vi "Generate Synchronous Strings For Moving Motors.vi"(7 "Motor List":u8[](array[numeric]), 8 "Error in (no error)":errorcluster, 9 "Dynamixel Speeds":u16[][](array[numeric]), 11 "Dynamixel Positions":u16[][](array[numeric])) -> (0 "Error out":errorcluster, 3 "Compiled Sync Parameters":string[](array[string]))   [LabVIEW 2016]
doc: "This VI combines the <B>Motor List</B> and corresponding positions and speeds in to sychronous write command. These commands when issues will move all of the motors at the same time."
uses:
  <instrlib>/Dynamixel Motor/Dynamixel Motor.lvlib
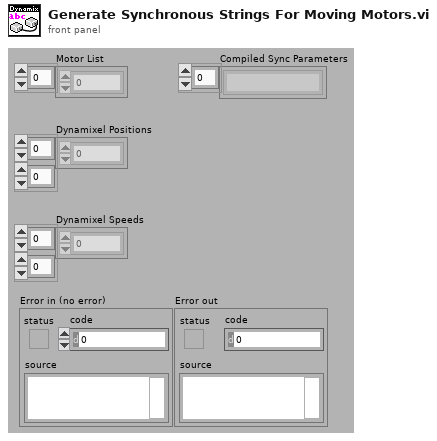
[diagram p1: front panel]
types:
  T1 = enum16{"big-endian, network order", "native, host order", "little-endian"}
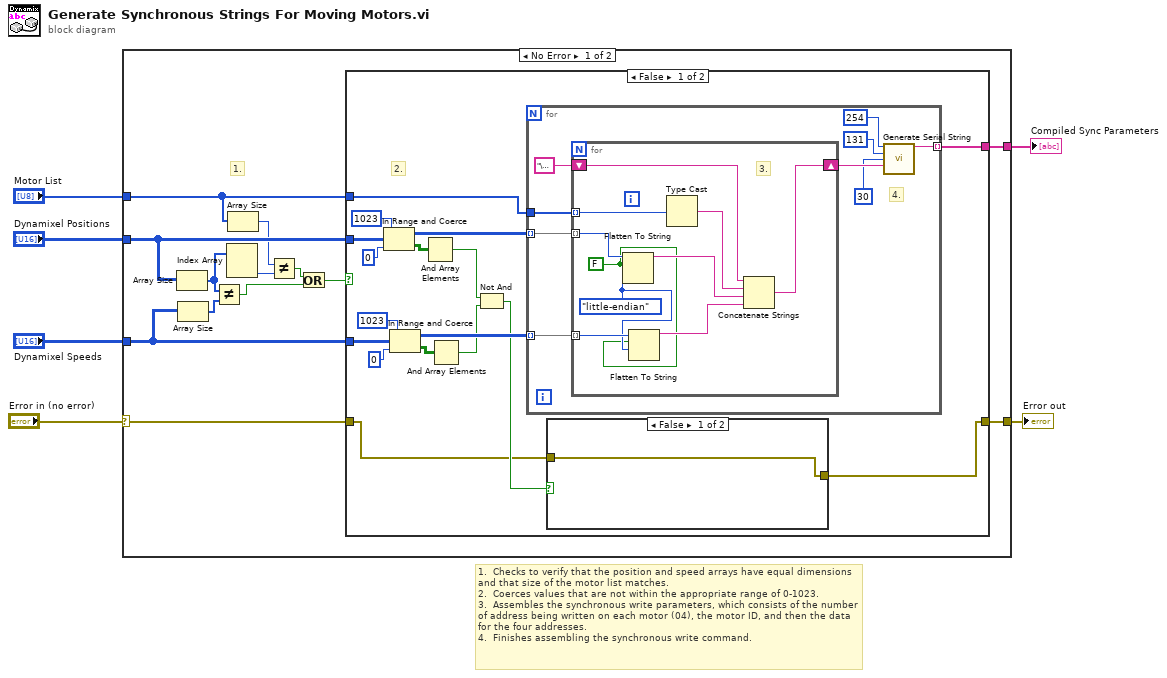
[diagram p0: block diagram]
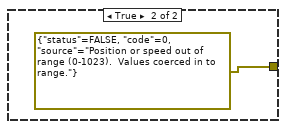
[diagram p2: hidden frame]
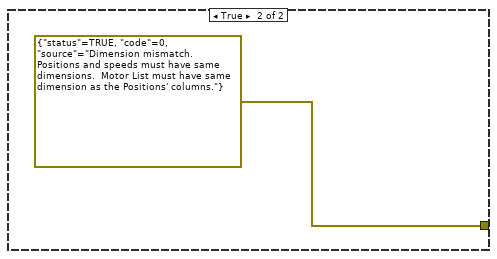
[diagram p3: hidden frame]
diagram:
  # "1.  Checks to verify that the position and speed arrays have equal dimensions \nand that size of the motor list matches.\n2.  Coerces values that are not within the appropriate range of 0-1023.\n3.  Assembles the synchronous write parameters, which consists of the number \nof address being written on each motor (04), the motor ID, and then the data \nfor the four addresses.\n4.  Finishes assembling the synchronous write command."
  n1 = case shown="No Error" "Error in (no error)" {
    selector: "Error in (no error)" -> [w7 w59]
    tunnel: [w19 _] -> w6
    tunnel: "Dynamixel Positions" -> [w18 _]
    tunnel: "Dynamixel Speeds" -> [w17 _]
    tunnel: "Motor List" -> [w15 _]
    tunnel: [w8 w59] -> w2
    frame No Error {
      # "1."
      n2 = Array Size(array=w18) -> (size(s)=w12:i32[])
      n3 = Array Size(array=w17) -> (size(s)=w16:i32[])
      n4 = Not Equal?(x=w12, y=w16) -> (x != y?=w13:bool)
      n5 = Index Array(array=w12) -> (element #2=w9:i32)  [unwired: 2 in, 1 out]
      n6 = Array Size(array=w15) -> (size(s)=w10:i32)
      n7 = Not Equal?(x=w10, y=w9) -> (x != y?=w11:bool)
      n8 = Or(x=w11, y=w13) -> (x .or. y?=w14:bool)
      n9 = case shown="False" w14 {
        tunnel: [w36 _] -> w19
        tunnel: w18 -> [w29 _]
        tunnel: w17 -> [w28 _]
        tunnel: w15 -> [w27 _]
        tunnel: [w20 errorcluster {"status"=TRUE, "code"=0, "source"="Dimension mismatch.  Positions and speeds must have same dimensions.  Motor List must have same dimension as the Positions' columns."} ("error in (no error)")] -> w8
        tunnel: w7 -> [w21 _]
        frame False {
          # "2."
          n10 = In Range and Coerce(upper limit=u16 1023, x=w29, lower limit=u16 0) -> (coerced(x)=w33:u16[][], In Range?=w25:bool[][])
          n11 = In Range and Coerce(upper limit=u16 1023, x=w28, lower limit=u16 0) -> (coerced(x)=w30:u16[][], In Range?=w26:bool[][])
          n12 = And Array Elements(Boolean array=w25) -> (logical AND=w23:bool)
          n13 = And Array Elements(Boolean array=w26) -> (logical AND=w24:bool)
          n14 = Not And(1:w24, 2:w23) -> (0:w22:bool)
          n15 = for {
            tunnel: w33 -> [w47] mode=indexing
            tunnel: w30 -> [w46] mode=indexing
            tunnel: [w42] -> w36 mode=indexing
            tunnel: w27 -> [w44]
            # "4."
            n16 = for {
              tunnel: w47 -> [w53] mode=indexing
              tunnel: w46 -> [w51] mode=indexing
              shift-right: [w57] -> w43
              shift-left: "\u0004" -> [w56]
              tunnel: w44 -> [w55] mode=indexing
              w49 = T1."little-endian" ("byte order (0:big-endian, network order)")
              w48 = FALSE ("prepend array or string size? (T)")
              # "3."
              n17 = Flatten To String(anything=w53, prepend array or string size? (T)=w48, byte order (0:big-endian, network order)=w49) -> (data string=w52:string)  [unwired: 1 in, 2 out]
              n18 = Flatten To String(anything=w51, prepend array or string size? (T)=w48, byte order (0:big-endian, network order)=w49) -> (data string=w50:string)  [unwired: 1 in, 2 out]
              n19 = Type Cast(x=w55) -> (*(type *) &x=w54:string)  [unwired: 1 in]
              n20 = Concatenate Strings(w56, w54, w52, w50) -> (w57:string)
            }
            n21 = call <instrlib>:"Generate Serial String.vi"("Motor ID"=u8 254 ("Motor ID (0)"), "Command"=u8 131 ("Motor ID (0)"), "Address"=u8 30 ("Motor ID (0)"), "Parameters"=w43) -> ("Command to Serial"=w42:string)  [unwired: 10 in, 1 out]
          }
          n22 = case shown="False" w22 {
            tunnel: w21 -> [w37 _]
            tunnel: [w37 errorcluster {"status"=FALSE, "code"=0, "source"="Position or speed out of range (0-1023).  Values coerced in to range."} ("error in (no error)")] -> w20
            frame False {
            }
            frame True {
            }
          }
        }
        frame True {
        }
      }
    }
    frame Error {
    }
  }
  "Compiled Sync Parameters" <- w6
  "Error out" <- w2
